vi "Tetra_ESN-NoCheck.vi"(0 "COMPORT":refnum<visa-resource-name>="COM4", 1 "BC_Esn":string, 11 "error in (no error)":errorcluster, 12 "DoEsnMatch(t)":bool, 13 "Open Ser(t)":bool, 14 "Close Ser(t)":bool) -> (2 "esn_match?(t)":bool, 3 "read":string="#Family: 0x2D\n#Serial: 0x000036092740\r\n", 4 "comport":refnum<visa-resource-name>="COM4", 8 "esn":string, 15 "error out":errorcluster)   [LabVIEW 2018]
doc: "This example performs writes and reads on a serial port, as directed by the user. You can press the Write and Read buttons, and change the Read Count, while the example is running.\n\nThe parameters set for the serial port must match the parameters of the connected instrument or device. In this example, the Read Count parameter specifies the number of bytes that the serial port reads. If there were more bytes at the port than the specified number, those bytes would not be read. If there were less bytes at the port than the specified number, you would receive a timeout error.\n\nThis example expands upon the flow control options for XON and XOFF, allowing the user to choose those control characters. Also, the user can enable or disable a termination character. Some devices require a termination character in order to identify the end of command strings. Some devices send a termination character to signify the end of data to be read. This example shows how you can end the Read operation once a termination character is detected in the buffer and/or append a termination character at the end of the Write data."
panel:
  out "VI Name":string
  out "Success":bool
  # "0xA is equivalent to a '\\n' character, which is a line feed."
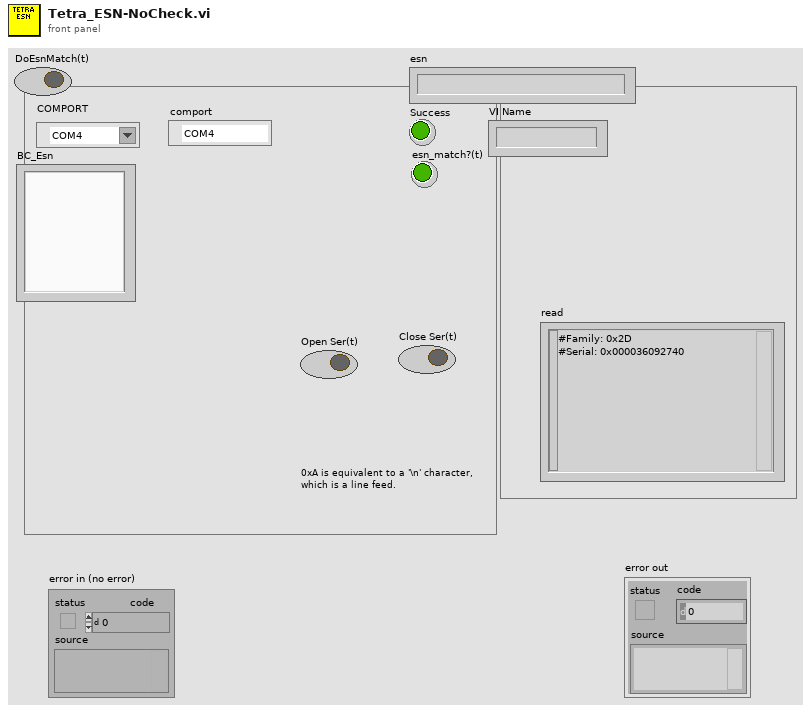
[diagram p1: front panel]
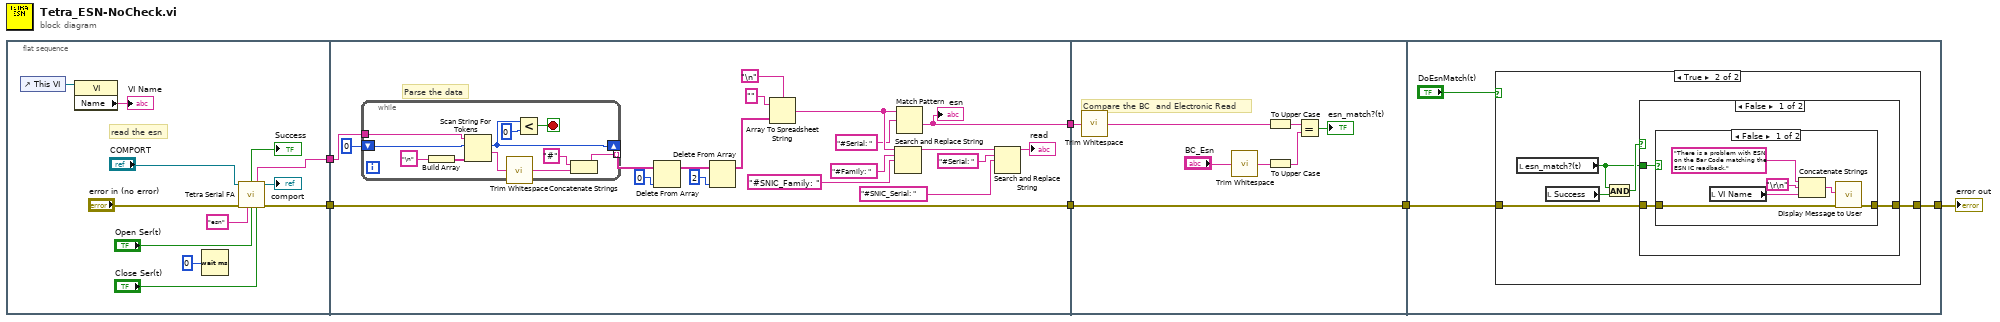
[diagram p0: block diagram]
diagram:
  n1 = flat-sequence {
    tunnel: [w12] -> w6
    tunnel: [w9] -> w2
    tunnel: w6 -> [w22]
    tunnel: [w20] -> w5
    tunnel: w2 -> [w19]
    tunnel: [w19] -> w1
    tunnel: w5 -> [w56]
    tunnel: [w51] -> w3
    tunnel: w1 -> [w51]
    tunnel: [w59] -> w4
    tunnel: w3 -> [w58]
    frame #0 {
      # "read the esn"
      n2 = control-ref of="This VI"() -> (w7:refnum<vi>)
      n3 = property class="VI"(reference=w7) -> ("Name"=→"VI Name":string)  [unwired: 1 in, 2 out]
      n4 = Wait (ms)(milliseconds to wait=u32 0) -> ()  [unwired: 1 out]
      n5 = call "Tetra Serial FA.vi"("COMPORT"="COMPORT", "error in (no error)"="error in (no error)", "Command"="esn", "Open Ser(t)"="Open Ser(t)", "Close Ser(t)"="Close Ser(t)") -> ("Success"=→"Success":bool, "output"=w12:string, "comport"=→"comport":refnum<visa-resource-name>, "error out"=w9:errorcluster)  [unwired: 7 in]
    }
    frame #1 {
      # "Parse the data"
      n6 = while {
        tunnel: [w39] -> w32 mode=indexing
        shift-right: [w46] -> _
        shift-left: 0 ("offset past token") -> [w45]
        tunnel: w22 -> [w43]
        stop <- w47 stop-if-true
        n7 = Build Array("\n") -> (w44:string[])
        n8 = Scan String For Tokens(6:w44, 8:w45, 9:w43) -> (1:w40:string, 2:w46:i32)  [unwired: 3 in, 2 out]
        n9 = call <vilib>:"Trim Whitespace.vi"("string"=w40) -> ("trimmed string"=w38:string)  [unwired: 1 in]
        n10 = Less?(x=w46, y=0) -> (x < y?=w47:bool)
        n11 = Concatenate Strings("#" ("string"), w38) -> (w39:string)
      }
      n12 = Delete From Array(array=w32, index=0) -> (array with subset deleted=w33:string[])  [unwired: 1 in, 1 out]
      n13 = Delete From Array(array=w33, index=2) -> (array with subset deleted=w34:string[])  [unwired: 1 in, 1 out]
      n14 = Array To Spreadsheet String(delimiter (Tab)="\n", array=w34, 3:"" ("format string")) -> (spreadsheet string=w36:string)
      n15 = Search and Replace String(input string=w36, search string="#Family: ", replace string="#SNIC_Family: " ("search string")) -> (result string=w35:string)  [unwired: 5 in, 3 out]
      n16 = Match Pattern(string=w36, regular expression="#Serial: ") -> (after substring=w20:string)  [unwired: 1 in, 3 out]
      "esn" <- w20
      n17 = Search and Replace String(input string=w35, search string="#Serial: ", replace string="#SNIC_Serial: " ("search string")) -> (result string=→"read":string)  [unwired: 5 in, 3 out]
    }
    frame #2 {
      # "Compare the BC  and Electronic Read"
      n18 = call <vilib>:"Trim Whitespace.vi"("string"=w56) -> ("trimmed string"=w52:string)  [unwired: 1 in]
      n19 = call <vilib>:"Trim Whitespace.vi"("string"="BC_Esn") -> ("trimmed string"=w53:string)  [unwired: 1 in]
      n20 = To Upper Case(1:w52) -> (0:w49:string)
      n21 = To Upper Case(1:w53) -> (0:w50:string)
      n22 = Equal?(x=w49, y=w50) -> (x = y?=→"esn_match?(t)":bool)
    }
    frame #3 {
      n23 = case shown="True" "DoEsnMatch(t)" {
        tunnel: [w60 w65] -> w59
        tunnel: w58 -> [w60 w64]
        frame False {
        }
        frame True {
          n24 = local read "esn_match?(t)"() -> (w61:bool)
          n25 = local read "Success"() -> (w62:bool)
          n26 = And(x=w61, y=w62) -> (x .and. y?=w63:bool)
          n27 = case shown="False" w63 {
            tunnel: [w67 w76] -> w65
            tunnel: w64 -> [w66 w76]
            tunnel: w61 -> [w68 _]
            frame False {
              n28 = case shown="False" w68 {
                tunnel: [w70 w75] -> w67
                tunnel: w66 -> [w69 w75]
                frame False {
                  n29 = local read "VI Name"() -> (w74:string)
                  n30 = Concatenate Strings("There is a problem with ESN on the Bar Code matching the ESN IC readback." ("Message"), "\r\n", w74) -> (w73:string)
                  n31 = call "Display Message to User"("error in (no error)"=w69, "Message"=w73) -> ("error out"=w70:errorcluster)  [unwired: 8 in, 1 out]
                }
                frame True {
                }
              }
            }
            frame True {
            }
          }
        }
      }
    }
  }
  "error out" <- w4
